vi "Check Inhibit.vi"(8 "error in (no error)":errorcluster, 11 "2WayValveV in":refnum<class "2WayValveV.lvclass">) -> (0 "error out":errorcluster, 3 "2WayValveV out":refnum<class "2WayValveV.lvclass">)   [LabVIEW 2020, in "VolatusGUIElements.lvlib" / "2WayValveV.lvclass"]
uses:
  2WayValveV.lvclass
  2WayValveV.lvclass/2WayValveV.ctl
  lv-vecto/Vecto/Channel DBL/Channel DBL.lvclass
  lv-vecto/Vecto/Vecto.lvlib
  VolatusGUI/GUI Element/GUI Element.lvclass
  C:/dev/lv20CE/relink/lv-volatus/VolatusGUI/GUI Element/GUI Element.lvclass
  C:/dev/lv20CE/relink/lv-volatus/VolatusGUIElements/2WayValveV/2WayValveV.lvclass
  C:/dev/lv20CE/relink/lv-volatus/VolatusGUI/OnValueChangeHandler/OnValueChangeHandler.lvclass
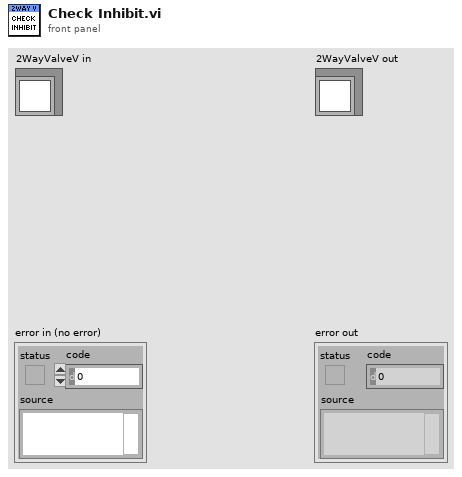
[diagram p1: front panel]
types:
  T1 = enum8{"Enabled", "Disabled", "Disabled and Grayed Out"}
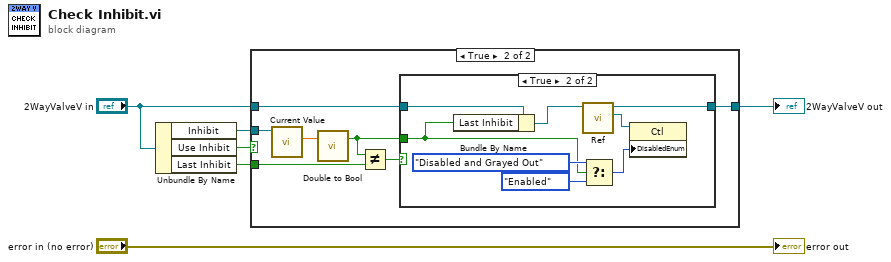
[diagram p0: block diagram]
diagram:
  n1 = Unbundle By Name("2WayValveV in") -> ("Inhibit"=w4:refnum<class "Channel DBL.lvclass">, "Use Inhibit"=w5:bool, "Last Inhibit"=w3:bool)
  n2 = case shown="True" w5 {
    tunnel: w4 -> [_ w14]
    tunnel: w3 -> [_ w12]
    tunnel: "2WayValveV in" -> [w7 w9]
    tunnel: [w7 w8] -> w1
    frame False {
    }
    frame True {
      n3 = call "Current Value.vi"("Channel in"=w14) -> ("Scaled"=w13:dbl)  [unwired: 6 in, 4 out]
      n4 = call "Double to Bool.vi"("Double"=w13) -> ("Bool"=w10:bool)  [unwired: 2 in]
      n5 = Not Equal?(x=w10, y=w12) -> (x != y?=w11:bool)
      n6 = case shown="True" w11 {
        tunnel: w10 -> [_ w16]
        tunnel: w9 -> [w15 w23]
        tunnel: [w15 w21] -> w8
        frame False {
        }
        frame True {
          n7 = Bundle By Name(cluster=w23, "Last Inhibit"=w16) -> (w17:refnum<class "2WayValveV.lvclass">)
          n8 = call "Ref.vi"("GUI Element in"=w17) -> ("Ref"=w22:refnum<vi>, "GUI Element out"=w21:refnum<class "2WayValveV.lvclass">)  [unwired: 9 in]
          n9 = Select(t=T1."Disabled and Grayed Out" ("Disabled"), s=w16, f=T1."Enabled" ("Disabled")) -> (s? t:f=w18:T1)
          n10 = property class="Ctl"(reference=w22, "DisabledEnum"=w18) -> ()  [unwired: 1 in, 2 out]
        }
      }
    }
  }
  "2WayValveV out" <- w1
  "error out" <- "error in (no error)"
